vi "LPS22HH DUT config.vi"(6 "error in":errorcluster, 9 "resource name":refnum<k15>="PXI1Slot2,PXI1Slot3") -> (0 "error out":errorcluster, 3 "instrument handle out":refnum<k15>)   [LabVIEW 2023, in "LPS22Demo.lvlib"]
uses:
  LPS22Demo.lvlib
  <instrlib>/niDigital/niDigital.llb/niDigital Load Specifications Levels and Timing (Single).vi
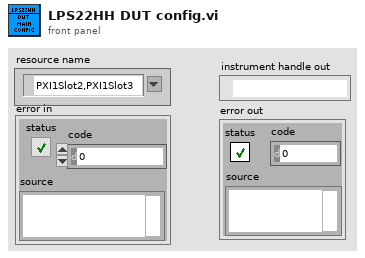
[diagram p1: front panel]
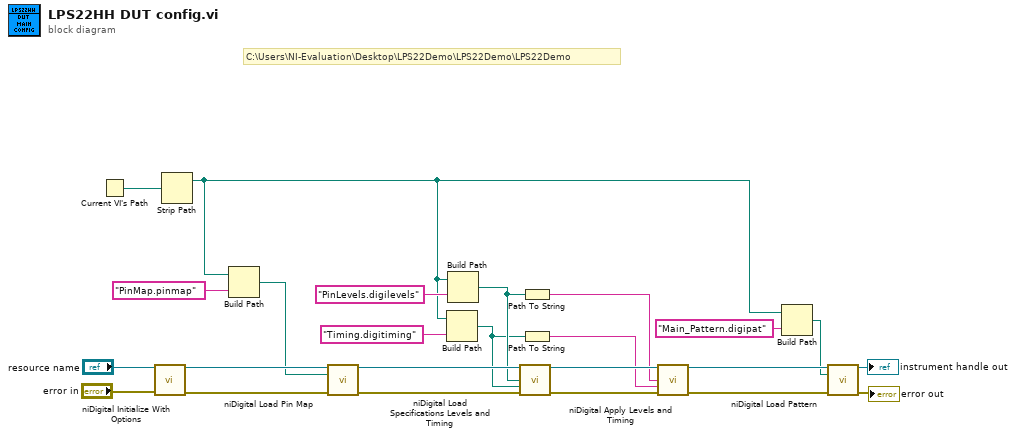
[diagram p0: block diagram]
diagram:
  # "C:\\Users\\NI-Evaluation\\Desktop\\LPS22Demo\\LPS22Demo\\LPS22Demo"
  n1 = Current VI's Path() -> (path=w10:path)
  n2 = call <instrlib>:"niDigital Initialize With Options.vi"("resource name"="resource name", "error in"="error in") -> ("instrument handle"=w20:refnum<k15>, "error out"=w19:errorcluster)  [unwired: 12 in]
  n3 = Strip Path(path=w10) -> (stripped path=w1:path)  [unwired: 1 out]
  n4 = Build Path(base path=w1, name or relative path="PinMap.pinmap") -> (appended path=w8:path)
  n5 = call <instrlib>:"niDigital Load Pin Map.vi"("instrument handle"=w20, "pin map file"=w8, "error in"=w19) -> ("instrument handle out"=w18:refnum<k15>, "error out"=w17:errorcluster)  [unwired: 11 in]
  n6 = Build Path(base path=w1, name or relative path="Timing.digitiming") -> (appended path=w2:path)
  n7 = Build Path(base path=w1, name or relative path="PinLevels.digilevels") -> (appended path=w3:path)
  n8 = call-poly <instrlib>:"niDigital Load Specifications Levels and Timing.vi"("instrument handle"=w18, "levels file path"=w3, "timing file path"=w2, "error in"=w17) -> ("instrument handle out"=w24:refnum<k15>, "error out"=w23:errorcluster)  [unwired: 10 in]
  n9 = Path To String(path=w3) -> (string=w16:string)
  n10 = Path To String(path=w2) -> (string=w15:string)
  n11 = call <instrlib>:"niDigital Apply Levels and Timing.vi"("instrument handle"=w24, "levels sheet"=w16, "timing sheet"=w15, "error in"=w23) -> ("instrument handle out"=w21:refnum<k15>, "error out"=w22:errorcluster)  [unwired: 10 in]
  n12 = Build Path(base path=w1, name or relative path="Main_Pattern.digipat") -> (appended path=w4:path)
  n13 = call <instrlib>:"niDigital Load Pattern.vi"("instrument handle"=w21, "pattern file"=w4, "error in"=w22) -> ("instrument handle out"=→"instrument handle out":refnum<k15>, "error out"=→"error out":errorcluster)  [unwired: 11 in]
